vi "Database_MLFB_Delete.vi"(3 "error in":errorcluster, 4 "Language":T2, 5 "MLFB":string, 6 "connection reference":T1) -> (0 "error out":errorcluster, 1 "Message":string, 2 "connection reference out":T1)   [LabVIEW 2015]
uses:
  CustomControl/Lang_Control.ctl
  <vilib>/addons/database/Connection.llb/Conn ObjectReference.ctl
  <vilib>/addons/database/NI_Database_API.lvlib
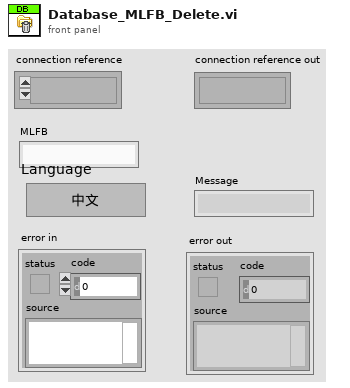
[diagram p1: front panel]
types:
  T1 = typedef "NI_Database_API.lvlib/Conn ObjectReference.ctl" = refnum<k1>
  T2 = typedef "Lang_Control.ctl" = enum16{"中文", "English"}
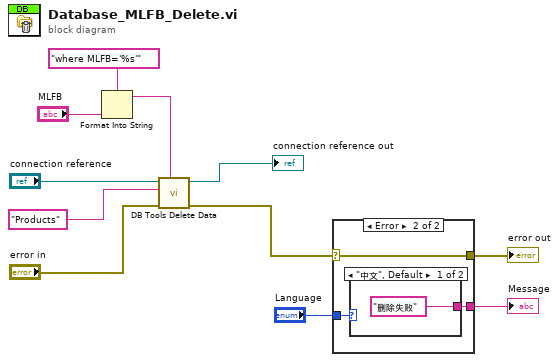
[diagram p0: block diagram]
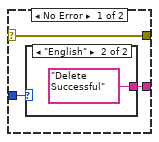
[diagram p2: hidden frame]
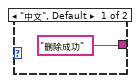
[diagram p3: hidden frame]
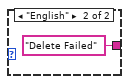
[diagram p4: hidden frame]
diagram:
  n1 = Format Into String(format string="where MLFB='%s'", "MLFB") -> (resulting string=w7:string)  [unwired: 2 in, 1 out]
  n2 = call <vilib>:"DB Tools Delete Data.vi"("condition"=w7, "error in (no error)"="error in", "table"="Products", "connection reference"="connection reference") -> ("error out"=w4:errorcluster, "connection reference out"=→"connection reference out":T1)  [unwired: 6 in]
  n3 = case shown="Error" w4 {
    selector: w4 -> [w14 w19]
    tunnel: [w14 w19] -> w11
    tunnel: "Language" -> [w13 w18]
    tunnel: [w12 w17] -> w8
    frame No Error {
      n4 = case shown="\"English\"" w13 {
        tunnel: ["删除成功" "Delete Successful"] -> w12
        frame "中文", Default {
        }
        frame "English" {
        }
      }
    }
    frame Error {
      n5 = case shown="\"中文\", Default" w18 {
        tunnel: ["删除失败" "Delete Failed"] -> w17
        frame "中文", Default {
        }
        frame "English" {
        }
      }
    }
  }
  "error out" <- w11
  "Message" <- w8
